vi "FWHM.vi"(4 "ntimes":i32=5, 5 "method":i32(ring)=3 items=["nearest", "bilinear", "bicubic", "bicubic spline"], 6 "error in (no error)":errorcluster, 9 "USB4000 In":T1) -> (0 "error out":errorcluster, 1 "Spectral Interpolated":T2, 2 "Spectral Raw":T2, 3 "USB4000 Out":T1)   [LabVIEW 2012]
uses:
  Controls/USB4000_Data.ctl
  <vilib>/gmath/NI_Gmath.lvlib
panel:
  out "Peak WL":dbl
  in  "Index":i32=850
  in  "EL Intensity":dbl[](array[numeric])
  in  "Lambda":dbl[](array[numeric])
  out "CWl Interpolated":dbl
  out "CWl Raw":dbl
  out "FWHM Raw":dbl
  out "FWHM Interpolated":dbl
  out "yi":dbl[](array[numeric]) format="%_6g"
  out "xi used":dbl[](array[numeric]) format="%_6g"
  out "Spect Interpolated":cluster{"RB Arr":dbl[], "RB Spect Arr":dbl[]}[](graph)
  out "Spect Raw":cluster{"all rows":dbl[], "all rows":dbl[]}[](graph)
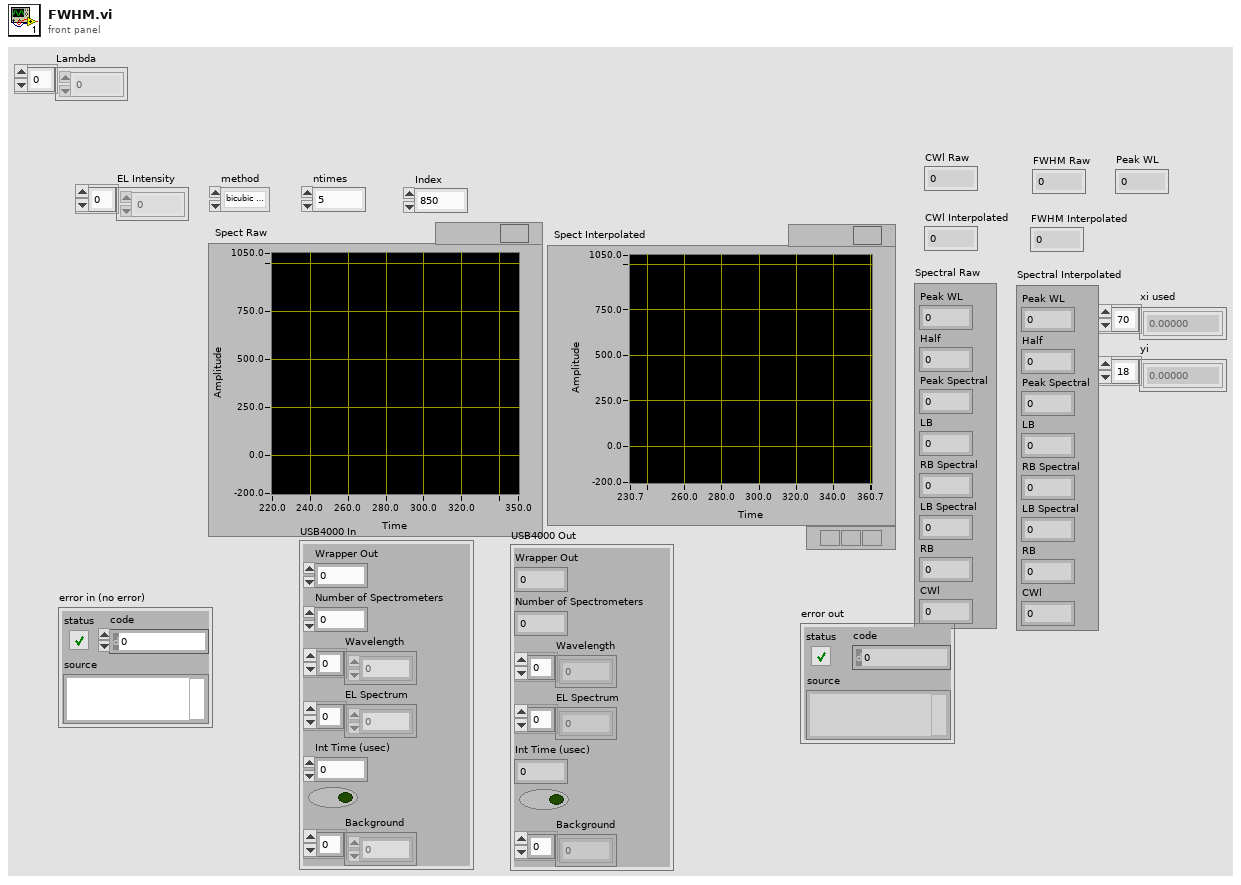
[diagram p1: front panel]
types:
  T1 = typedef "USB4000_Data.ctl" = cluster{"Wrapper Out":u32, "Number of Spectrometers":i32, "Wavelength":dbl[], "EL Spectrum":dbl[], "Int Time (usec)":i32, bool, "Background":dbl[]}
  T2 = cluster{"Peak WL":dbl, "Half":dbl, "Peak Spectral":dbl, "LB":dbl, "RB Spectral":dbl, "LB Spectral":dbl, "RB":dbl, "CWl":dbl}
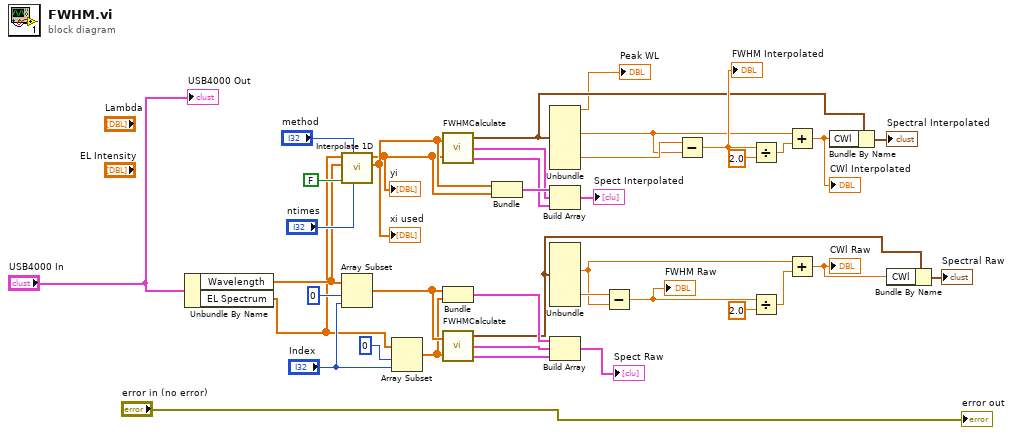
[diagram p0: block diagram]
diagram:
  n1 = Unbundle By Name("USB4000 In") -> ("Wavelength"=w4:dbl[], "EL Spectrum"=w3:dbl[])
  n2 = call <vilib>:"Interpolate 1D.vi"("ntimes"="ntimes", "method"="method", "X is monotonic"=FALSE, "X"=w4, "Y"=w3) -> ("xi used"=w34:dbl[], "yi"=w33:dbl[])  [unwired: 4 in, 1 out]
  "xi used" <- w34
  "yi" <- w33
  n3 = Array Subset "Array Subset"(array=w4, index=0, length="Index") -> (w8:dbl[])
  n4 = Array Subset(array=w3, index=0, length="Index") -> (w7:dbl[])
  n5 = call "FWHMCalculate.vi"("Lambda"=w34, "Spectra"=w33) -> ("Spectral Results"=w12:T2, "Right Band"=w30:cluster{dbl[], dbl[]}, "Left Band"=w29:cluster{dbl[], dbl[]})
  n6 = Bundle(w8, w7) -> (w38:cluster{dbl[], dbl[]})  [unwired: 1 in]
  n7 = call "FWHMCalculate.vi"("Lambda"=w8, "Spectra"=w7) -> ("Spectral Results"=w16:T2, "Right Band"=w28:cluster{dbl[], dbl[]}, "Left Band"=w27:cluster{dbl[], dbl[]})
  n8 = Bundle("xi used"=w34, "yi"=w33) -> (w32:cluster{"xi used":dbl[], "yi":dbl[]})  [unwired: 1 in]
  n9 = Unbundle(w12) -> ("Peak WL"=→"Peak WL":dbl, "LB"=w19:dbl, "RB"=w26:dbl)  [unwired: 5 out]
  n10 = Build Array(w32, w30, w29) -> (→"Spect Interpolated":cluster{"xi used":dbl[], "yi":dbl[]}[])
  n11 = Unbundle(w16) -> ("LB"=w17:dbl, "RB"=w25:dbl)  [unwired: 6 out]
  n12 = Build Array(w38, w28, w27) -> (→"Spect Raw":cluster{dbl[], dbl[]}[])
  n13 = Subtract(x=w25, y=w17) -> (x-y=w24:dbl)
  "FWHM Raw" <- w24
  n14 = Subtract(x=w26, y=w19) -> (x-y=w21:dbl)
  "FWHM Interpolated" <- w21
  n15 = Divide(x=w21, y=2.0) -> (x/y=w20:dbl)
  n16 = Divide(x=w24, y=2.0) -> (x/y=w18:dbl)
  n17 = Add(x=w19, y=w20) -> (x+y=w13:dbl)
  "CWl Interpolated" <- w13
  n18 = Add(x=w17, y=w18) -> (x+y=w15:dbl)
  "CWl Raw" <- w15
  n19 = Bundle By Name(cluster=w12, "CWl"=w13) -> (→"Spectral Interpolated":T2)
  n20 = Bundle By Name(cluster=w16, "CWl"=w15) -> (→"Spectral Raw":T2)
  "USB4000 Out" <- "USB4000 In"
  "error out" <- "error in (no error)"
